vi "Open File.vi"(7 "R/W":string="W", 10 "File ID":string, 11 "仪器地址":u32) -> (3 "OutPut":string)   [LabVIEW 2010, in "DCP551.lvlib"]
uses:
  DCP551.lvlib
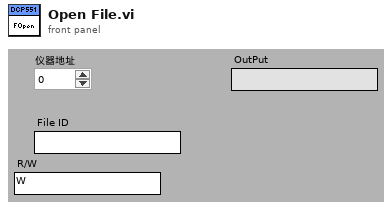
[diagram p1: front panel]
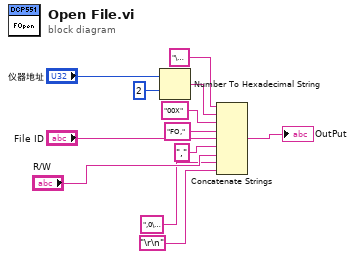
[diagram p0: block diagram]
diagram:
  n1 = Number To Hexadecimal String(1:i16 2 ("width (-)"), 2:"仪器地址") -> (0:w10:string)
  n2 = Concatenate Strings("\u0002" ("string"), w10, "00X" ("string"), "FO," ("string"), "File ID", "," ("string"), "R/W", ",0\u0003" ("string"), "\r\n") -> (→"OutPut":string)
